vi "GetLibraryVariable.vi"(3 "Parameter":string="H5T_STD_I8BE_g", 9 "error in (no error)":errorcluster) -> (0 "Value":i32, 6 "error out":errorcluster)   [LabVIEW 2009]
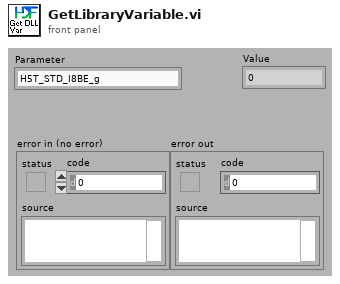
[diagram p1: front panel]
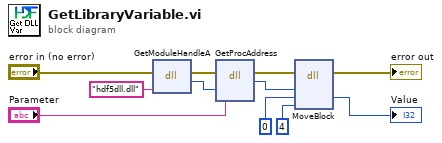
[diagram p0: block diagram]
diagram:
  n1 = dll-call lib="kernel32" fn="GetModuleHandleA"(error in="error in (no error)", "lpModuleName"="hdf5dll.dll") -> (error out=w11:errorcluster, "return type"=w10:i64)  [unwired: 3 in, 1 out]
  n2 = dll-call lib="kernel32" fn="GetProcAddress"(error in=w11, "hModule"=w10, "lpProcName"="Parameter") -> (error out=w9:errorcluster, "return type"=w7:i64)  [unwired: 4 in, 1 out]
  n3 = dll-call lib="LabVIEW" fn="MoveBlock"(error in=w9, "Address (Pointer)"=w7, "destination"=0 ("Size"), "size"=4 ("Size")) -> (error out=→"error out":errorcluster, "destination"=→"Value":i32)  [unwired: 5 in, 1 out]
